vi "detectFaults.vi"(8 "ErrorIn":errorcluster, 10 "Orders and indicators":T1[](array[typedef]), 11 "Fault Indicators":T7) -> (0 "ErrorOut":errorcluster, 3 "Fault detections":T2)   [LabVIEW 2019]
uses:
  calculateFaultIndicatorsVIs/FaultIndicators.ctl
  calculateFaultIndicatorsVIs/FaultDetections.ctl
  calculateFaultIndicatorsVIs/ParameterFaultDetection.ctl
  calculateFaultIndicatorsVIs/FaultParameter.ctl
  calculateFaultIndicatorsVIs/FrequencyFaultDetection.ctl
  calculateFaultIndicatorsVIs/OrdersFaultDetection.ctl
  OrderAndIndicators.ctl
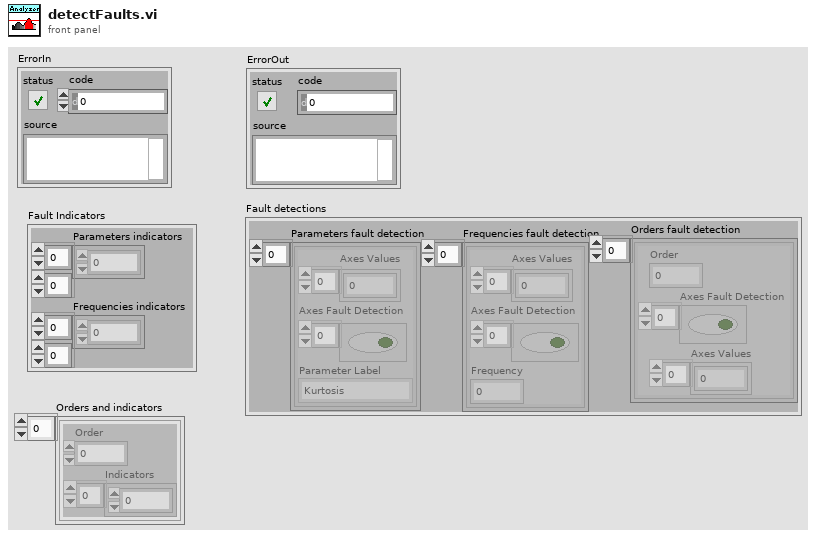
[diagram p1: front panel]
types:
  T1 = typedef "OrderAndIndicators.ctl" = cluster{"Order":dbl, "Indicators":dbl[]}
  T2 = typedef "FaultDetections.ctl" = cluster{"Parameters fault detection":T3[], "Frequencies fault detection":T5[], "Orders fault detection":T6[]}
  T3 = typedef "ParameterFaultDetection.ctl" = cluster{"Axes Values":dbl[], "Axes Fault Detection":bool[], "Parameter Label":T4}
  T4 = typedef "FaultParameter.ctl" = enum16{"Kurtosis", "RMS", "Crest factor"}
  T5 = typedef "FrequencyFaultDetection.ctl" = cluster{"Axes Values":dbl[], "Axes Fault Detection":bool[], "Frequency":dbl}
  T6 = typedef "OrdersFaultDetection.ctl" = cluster{"Order":dbl, "Axes Fault Detection":bool[], "Axes Values":dbl[]}
  T7 = typedef "FaultIndicators.ctl" = cluster{"Parameters indicators":dbl[][], "Frequencies indicators":dbl[][]}
  T8 = typedef "AnalyzerSettings.ctl" = cluster{"Create NS Timeout Code":i32, "Destroy NS Timeout Code":i32, "All threads":T9[], "AnalysisSettings":T10}
  T9 = typedef "AThreads.ctl" = enum16{"UI", "analyzeAccelerationData", "aquireAccelerationData", "communicateWebServices", "TDMSmanager", "aquireTachoSignal"}
  T10 = typedef "AnalysisSettings.ctl" = cluster{"Fault Thresholds":T11, "Analysis series name":string, "Save data analysis?":bool, "Band size":i32, "OrderAnalysis?":bool, "Accelerometer":T12, "fs [Hz]":dbl, "Pulse per revolution":u16}
  T11 = typedef "Thresholds.ctl" = cluster{"Parameters labels":T4[], "Parameters thresholds":dbl[], "Freqs and thresholds":dbl[][], "Orders and thresholds":dbl[][]}
  T12 = typedef "Accelerometer.ctl" = enum16{"None", "MPU6050", "MMA7351"}
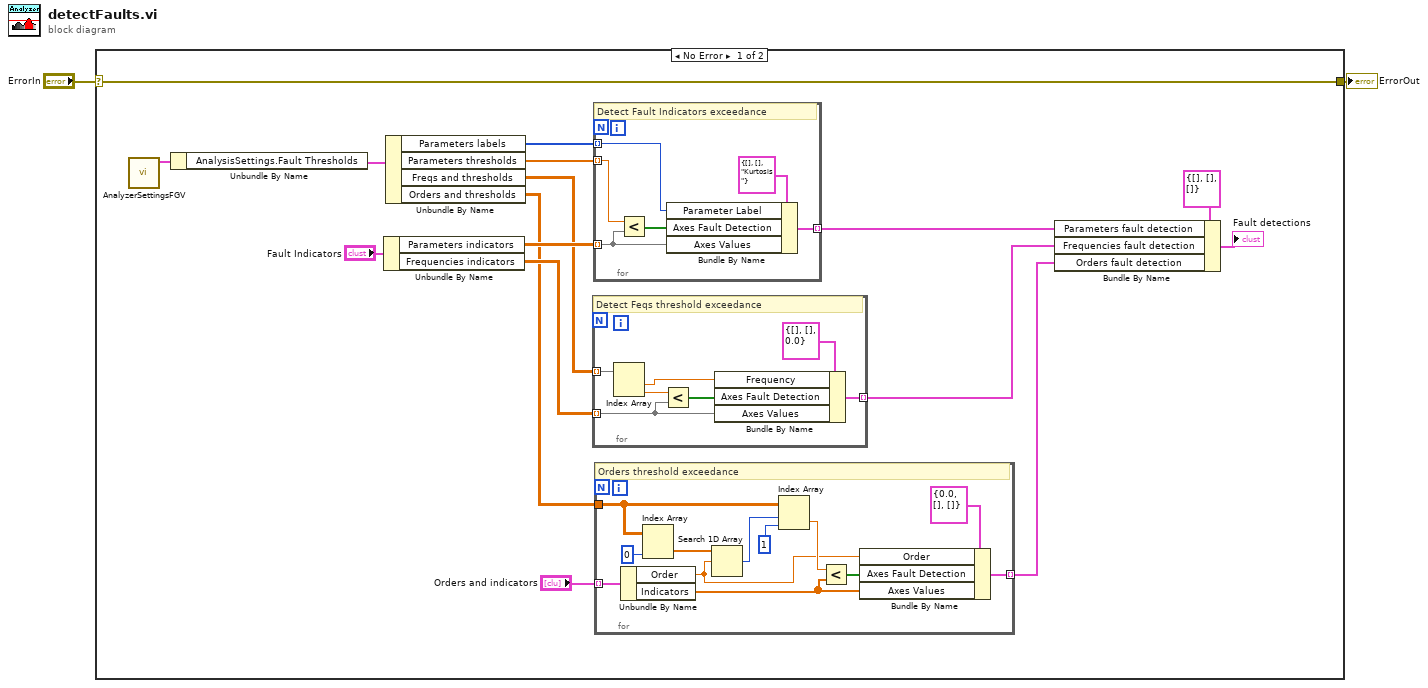
[diagram p0: block diagram]
diagram:
  n1 = case shown="No Error" "ErrorIn" {
    selector: "ErrorIn" -> [w6 w44]
    tunnel: [w6 w44] -> w1
    frame No Error {
      n2 = call "AnalyzerSettingsFGV.vi"() -> ("GlobalSettingsOut"=w15:T8)  [unwired: 11 in]
      n3 = Unbundle By Name(w15) -> ("AnalysisSettings.Fault Thresholds"=w14:T11)
      n4 = Unbundle By Name("Fault Indicators") -> ("Parameters indicators"=w18:dbl[][], "Frequencies indicators"=w17:dbl[][])
      n5 = Unbundle By Name(w14) -> ("Parameters labels"=w9:T4[], "Parameters thresholds"=w13:dbl[], "Freqs and thresholds"=w12:dbl[][], "Orders and thresholds"=w4:dbl[][])
      n6 = for {
        tunnel: w17 -> [w36] mode=indexing
        tunnel: w12 -> [w34] mode=indexing
        tunnel: [w35] -> w7 mode=indexing
        # "Detect Feqs threshold exceedance"
        n7 = Index Array(array=w34) -> (element #1=w31:dbl, element #2=w33:dbl)  [unwired: 2 in]
        n8 = Less?(x=w33, y=w36) -> (x < y?=w37:bool[])
        n9 = Bundle By Name(cluster=T5 {"Axes Values"=[], "Axes Fault Detection"=[], "Frequency"=0.0} ("AxesValueAndFaultDetection"), "Frequency"=w31, "Axes Fault Detection"=w37, "Axes Values"=w36) -> (w35:T5)
      }
      n10 = for {
        tunnel: w18 -> [w42] mode=indexing
        tunnel: w13 -> [w43] mode=indexing
        tunnel: [w40] -> w8 mode=indexing
        tunnel: w9 -> [w38] mode=indexing
        # "Detect Fault Indicators exceedance"
        n11 = Less?(x=w43, y=w42) -> (x < y?=w41:bool[])
        n12 = Bundle By Name(cluster=T3 {"Axes Values"=[], "Axes Fault Detection"=[], "Parameter Label"=enum."Kurtosis"} ("AxesValueAndFaultDetection"), "Parameter Label"=w38, "Axes Fault Detection"=w41, "Axes Values"=w42) -> (w40:T3)
      }
      n13 = for {
        tunnel: "Orders and indicators" -> [w30] mode=indexing
        tunnel: w4 -> [w27]
        tunnel: [w19] -> w3 mode=indexing
        # "Orders threshold exceedance"
        n14 = Unbundle By Name(w30) -> ("Order"=w20:dbl, "Indicators"=w21:dbl[])
        n15 = Index Array(array=w27, index (col)=0 ("disabled index (col)")) -> (element=w28:dbl[])  [unwired: 1 in]
        n16 = Search 1D Array(1D array=w28, element=w20) -> (index of element=w25:i32)  [unwired: 1 in]
        n17 = Index Array(array=w27, index (row)=w25, index (col)=1 ("disabled index (col)")) -> (element=w24:dbl)
        n18 = Less?(x=w24, y=w21) -> (x < y?=w22:bool[])
        n19 = Bundle By Name(cluster=T6 {"Order"=0.0, "Axes Fault Detection"=[], "Axes Values"=[]} ("Orders fault detection"), "Order"=w20, "Axes Fault Detection"=w22, "Axes Values"=w21) -> (w19:T6)
      }
      n20 = Bundle By Name(cluster=T2 {"Parameters fault detection"=[], "Frequencies fault detection"=[], "Orders fault detection"=[]} ("Fault detections"), "Parameters fault detection"=w8, "Frequencies fault detection"=w7, "Orders fault detection"=w3) -> (→"Fault detections":T2)
    }
    frame Error {
    }
  }
  "ErrorOut" <- w1
